vi "Get Data from FIFO (I16).vi"(7 "FIFO In":refnum<k21>="FIFOtoFFTLoop", 8 "Get New Data":bool, 11 "FFT State Info":T1) -> (0 "Data Valid":bool, 2 "Data":fxp<+,16,1>, 3 "FFT State Info Out":T1)   [LabVIEW 2011]
uses:
  <vilib>/rvi/DataTransferAndStorage/Container/Common/niFpgaContainerExecOnDevCompGetState.vi
  <vilib>/rvi/FIFO/Fifo_Resource/nirvififoEmulationSetSize.vi
  <vilib>/rvi/DataTransferAndStorage/Container/Common/niFpgaContainerGetUniqueNameForEmu.vi
  <vilib>/rvi/interface/RandomDataEmulation/nirviRandomDataFPGAFIFO.vi
  <vilib>/rvi/interface/RandomDataEmulation/niFpgaRandomDataHandleErrors.vi
  <vilib>/rvi/eio/common/nirviEmuReportErrorAndStop.vi
  <vilib>/rvi/FXPMathLib/basic elements/FxpDiscreteDelay/XNode/nifxpmath_DiscreteDelay.xnode
  <vilib>/rvi/DataTransferAndStorage/Container/XNode/niFpgaContainer.xnode
  <vilib>/rvi/FIFO/Fifo_Resource/niFpgaFifoEmulationRefIn.vi
  <vilib>/rvi/FXPMathLib/FxpInterpret/XNode/nifxpmath_Interpret.xnode
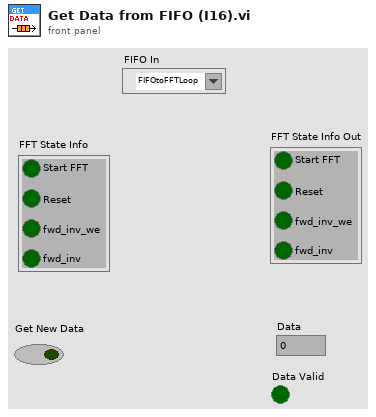
[diagram p1: front panel]
types:
  T1 = cluster{"Reset":bool, "Start FFT":bool, "fwd_inv_we":bool, "fwd_inv":bool}
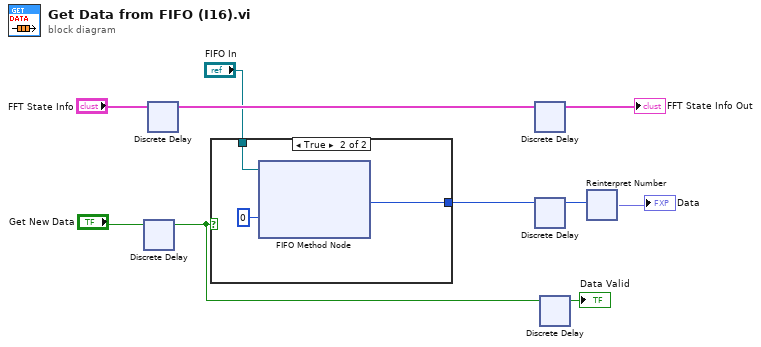
[diagram p0: block diagram]
diagram:
  n1 = xnode "Discrete Delay"("D"="Get New Data") -> ("Q"=w2:bool)
  n2 = xnode "Discrete Delay"("D"="FFT State Info") -> ("Q"=w8:T1)
  n3 = case shown="True" w2 {
    tunnel: [_ w11] -> w7
    tunnel: "FIFO In" -> [_ w13]
    frame False {
    }
    frame True {
      n4 = xnode ("FIFO Method Node")("Timeout"=0, "FIFO In"=w13) -> ("Element"=w11:i16)  [unwired: 2 out]
    }
  }
  n5 = xnode "Discrete Delay"("D"=w8) -> ("Q"=→"FFT State Info Out":T1)
  n6 = xnode "Discrete Delay"("D"=w7) -> ("Q"=w4:i16)
  n7 = xnode "Discrete Delay"("D"=w2) -> ("Q"=→"Data Valid":bool)
  n8 = xnode "Reinterpret Number"("x"=w4) -> ("y"=→"Data":fxp<+,16,1>)
